vi "1chHistogramRange (SubVI).vi"(6 "offset":i32, 10 "Histogram 1":u32[](array[numeric])) -> (2 "Output Range":T1)   [LabVIEW 2019]
doc: "c 2020 ReMiSYS All rights reserved."
panel:
  # "c 2020 ReMiSYS All rights reserved."
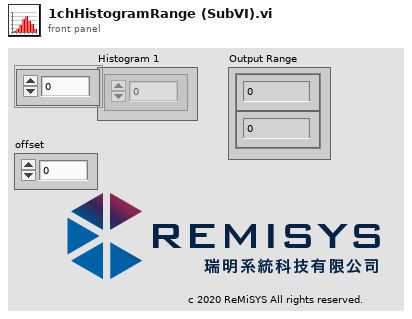
[diagram p1: front panel]
types:
  T1 = cluster{"Numeric Control":i32, "Numeric Control":i32}
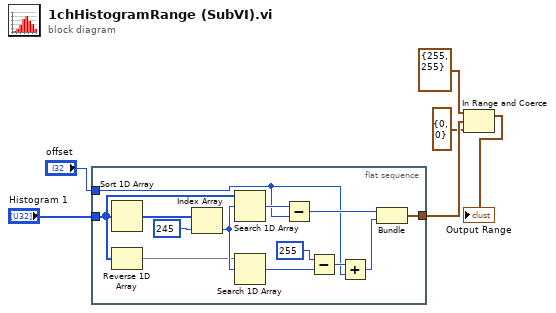
[diagram p0: block diagram]
diagram:
  n1 = flat-sequence {
    tunnel: "Histogram 1" -> [w16]
    tunnel: [w12] -> w4
    tunnel: "offset" -> [w7]
    frame #0 {
      n2 = Sort 1D Array(array=w16) -> (sorted array=w19:u32[])
      n3 = Reverse 1D Array(array=w16) -> (reversed array=w15:u32[])
      n4 = Index Array(array=w19, index=245) -> (element=w17:u32)
      n5 = Search 1D Array(1D array=w16, element=w17) -> (index of element=w11:i32)  [unwired: 1 in]
      n6 = Search 1D Array(1D array=w15, element=w17) -> (index of element=w14:i32)  [unwired: 1 in]
      n7 = Subtract(x=w11, y=w7) -> (x-y=w10:i32)
      n8 = Subtract(x=255, y=w14) -> (x-y=w9:i32)
      n9 = Add(x=w9, y=w7) -> (x+y=w8:i32)
      n10 = Bundle(w10, w8) -> (w12:cluster{i32, i32})  [unwired: 1 in]
    }
  }
  n11 = In Range and Coerce(upper limit=cluster{i32, i32} {255, 255}, x=w4, lower limit=cluster{i32, i32} {0, 0}) -> (coerced(x)=→"Output Range":cluster{i32, i32})  [unwired: 1 out]
